vi "FTW-JSON-Interpret-Timestamp.vi"(1 "JSON String":string) -> (0 "LabVIEW Timestamp":timestamp format="%<%Y-%m-%d %H:%M:%S%03u>T")   [LabVIEW 2015]
panel:
  # "Inputs"
  # "Outputs"
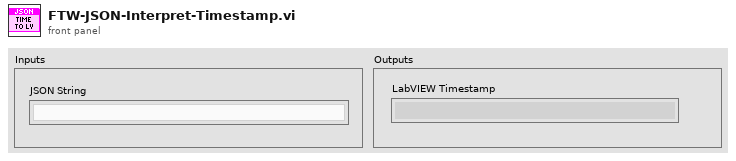
[diagram p1: front panel]
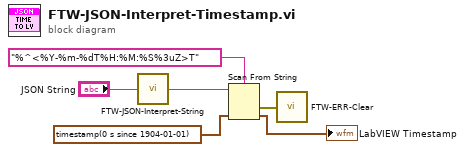
[diagram p0: block diagram]
diagram:
  n1 = call "FTW-JSON-Interpret-String.vi"("JSON String"="JSON String") -> ("LabVIEW String"=w2:string)
  n2 = Scan From String(format string="%^<%Y-%m-%dT%H:%M:%S%3uZ>T", input string=w2, default 1=timestamp(0 s since 1904-01-01) ("LabVIEW Timestamp")) -> (error out=w6:errorcluster, output 1=→"LabVIEW Timestamp":timestamp)  [unwired: 2 in, 2 out]
  n3 = call "FTW-ERR-Clear.vi"("error to snuff"=w6) -> ()  [unwired: 1 out]
